vi "ProcessBufferUpdates.vi"(11 "MockDisplacementSettings":T1={"SerialPort"="Slot3\\Port1", "BufferUpdateFIFO"="MockDisplacementCommandFIFO", "DisplacementMemory"="DisplacementMemory"}) -> ()   [LabVIEW 2016, in "FPGAMockDisplacement.lvlib"]
uses:
  FPGAMockDisplacement.lvlib
  DataTypes/MockDisplacementSettings.ctl
  <vilib>/rvi/Emulation/niFpgaGetClockAttributes.vi
  <vilib>/rvi/Emulation/niFpgaSctlEmulationGetInTimedLoop.vi
  <vilib>/rvi/Emulation/niFpgaEmulationReportErrorSimple.vi
  <vilib>/rvi/DataTransferAndStorage/Container/Common/niFpgaContainerExecOnDevCompGetState.vi
  <vilib>/rvi/Emulation/niFpgaEmulationIsFPGAContextNoSignature.vi
  <vilib>/rvi/errors/niFpgaSetErrorForExecOnDevCompSimple.vi
  <vilib>/rvi/eio/common/nirviEmuReportErrorAndStop.vi
  <vilib>/rvi/DataTransferAndStorage/Container/Common/niFpgaContainerGetUniqueNameForEmu.vi
  <vilib>/rvi/FIFO/Fifo_Resource/nirvififoEmulationSetSize.vi
  <vilib>/rvi/FIFO/Fifo_Resource/nirviFifoEmulationQueueMgr.vi
  <instcachedir>/0/nirviFifoEmulationQueueMgr_E5CAEC123FF24DC58D834DCA3CDAA9B5.lvgen/nirviFifoEmulationQueueMgr_E5CAEC123FF24DC58D834DCA3CDAA9B5_009.vi
  <vilib>/rvi/FIFO/Fifo_Resource/nirvififoEmulationDetermineInputValidOut.vi
  <vilib>/rvi/FIFO/Fifo_Resource/nirvififoEmulationCreateLock.vi
  <vilib>/rvi/Emulation/niFpgaProcessEmulError.vi
  <vilib>/rvi/FIFO/Fifo_Resource/nirvififoEmulationObtainLock.vi
  <vilib>/rvi/FIFO/Fifo_Resource/nirvififoEmulationReleaseLock.vi
  <vilib>/rvi/occurrence/nirviWaitOnOccurrenceBase.vi
  <vilib>/rvi/errors/nirviReportUnexpectedCaseInternalError.vi
  <vilib>/rvi/errors/nirviReportUnexpectedCaseInternalError (U32).vi
  <vilib>/Utility/error.llb/Clear Errors.vi
  <vilib>/rvi/interface/RandomDataEmulation/niFpgaRandomDataHandleErrors.vi
  <vilib>/rvi/Memory/Memory_Emulation/niFpgaMemoryEmulationCacheClearOnFirstRun.vi
  <vilib>/rvi/Memory/Memory_Emulation/nirvimemoryEmulationManagerCache_MakeExclusive.vi
  <vilib>/rvi/Memory/Memory_Emulation/niFpgaMemoryEmulationValidateCache.vi
  <vilib>/rvi/Memory/Memory_Emulation/nirvimemoryEmulationManagerCache_InsertValue.vi
  <vilib>/rvi/Memory/Memory_Emulation/nirvimemoryEmulationManagerCache_ReleaseExclusive.vi
  <vilib>/rvi/Memory/Memory_Emulation/nirvimemoryEmulationManagerCache_GetValue.vi
  <vilib>/rvi/Memory/Memory_Emulation/nirvimemoryEmulationManagerCache_SetValue.vi
  <vilib>/rvi/Emulation/niFpgaSctlEmulationResourceMgr.vi
  <vilib>/rvi/Emulation/niFpgaCriticalErrorInLSC.vi
  <vilib>/rvi/DataTransferAndStorage/Container/XNode/niFpgaContainer.xnode
  <vilib>/rvi/FIFO/Fifo_Resource/niFpgaFifoEmulationRefIn.vi
  <vilib>/rvi/Memory/Memory_Emulation/niFpgaMemoryEmulationRefIn.vi
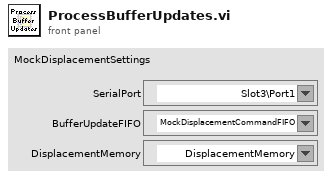
[diagram p1: front panel]
types:
  T1 = typedef "FPGAMockDisplacement.lvlib/MockDisplacementSettings.ctl" = cluster{"SerialPort":refnum<k21>, "BufferUpdateFIFO":refnum<k21>, "DisplacementMemory":refnum<k21>}
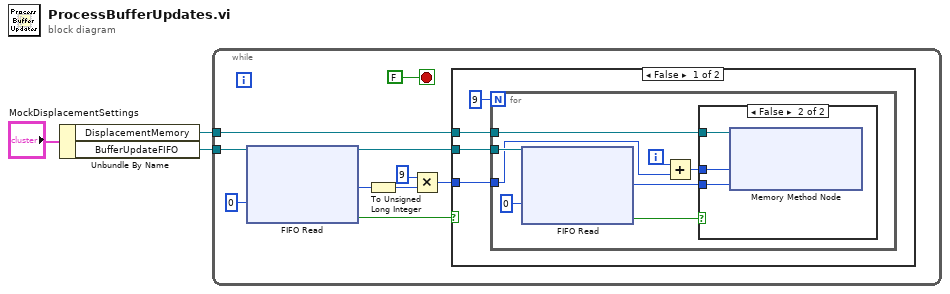
[diagram p0: block diagram]
diagram:
  n1 = Unbundle By Name("MockDisplacementSettings") -> ("DisplacementMemory"=w1:refnum<k21>, "BufferUpdateFIFO"=w2:refnum<k21>)
  n2 = while {
    tunnel: w2 -> [w12]
    tunnel: w1 -> [w8]
    stop <- FALSE stop-if-true
    n3 = xnode "FIFO Read"("Timeout"=0, "FIFO In"=w12) -> ("Element"=w9:u8, "Timed Out?"=w11:bool, "FIFO Out"=w10:refnum<k21>)
    n4 = To Unsigned Long Integer(number=w9) -> (unsigned 32bit integer=w6:u32)
    n5 = Multiply(x=u32 9, y=w6) -> (x*y=w4:u32)
    n6 = case shown="False" w11 {
      tunnel: w10 -> [w17 _]
      tunnel: w4 -> [w16 _]
      tunnel: w8 -> [w15 _]
      frame False {
        n7 = for {
          N: 9 -> [_]
          tunnel: w17 -> [w25]
          tunnel: w16 -> [w20]
          tunnel: w15 -> [w23]
          i -> [w18]
          n8 = xnode "FIFO Read"("Timeout"=0, "FIFO In"=w25) -> ("Element"=w22:u8, "Timed Out?"=w24:bool)  [unwired: 1 out]
          n9 = Add(x=w18, y=w20) -> (x+y=w21:u32)
          n10 = case shown="False" w24 {
            tunnel: w22 -> [_ w28]
            tunnel: w21 -> [_ w27]
            tunnel: w23 -> [_ w26]
            frame True {
            }
            frame False {
              n11 = xnode ("Memory Method Node")("Address"=w27, "Data"=w28, "Memory In"=w26) -> ()  [unwired: 1 out]
            }
          }
        }
      }
      frame True {
      }
    }
  }
